vi "Test Find Tests From lvlib.vi"(8 "error in (no error)":errorcluster, 11 "Test Case In":refnum<class "Test FInder Test.lvclass">) -> (0 "error out":errorcluster, 3 "Test Case Out":refnum<class "Test FInder Test.lvclass">)   [LabVIEW 2020, in "Test FInder Test.lvclass"]
uses:
  Test FInder Test.lvclass
  <vilib>/Astemes/LUnit/Test Case.lvclass/Test Case.ctl
  <vilib>/Astemes/LUnit/Core/LUnit Test Case/Private/Append Fail Result.vi
  <vilib>/Astemes/LUnit/Core/LUnit Test Case/Private/Append Pass Result.vi
  <vilib>/Astemes/LUnit/Core/LUnit Test Case/Private/Run In UI.vi
  <vilib>/Utility/error.llb/Clear Errors.vi
  Test FInder Test.lvclass/Test FInder Test.ctl
  source/Framework/Test Finder/Test Finder.lvclass
  source/LUnit Test Suite.lvclass
  80f47747-7e17-4ea4-8ca2-817b5c50055d.vi
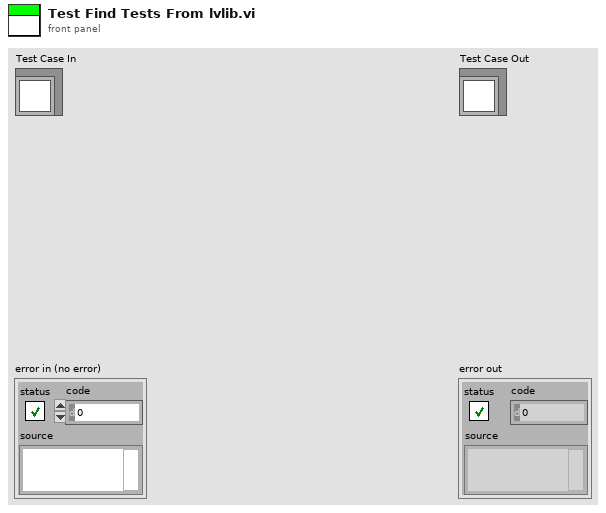
[diagram p1: front panel]
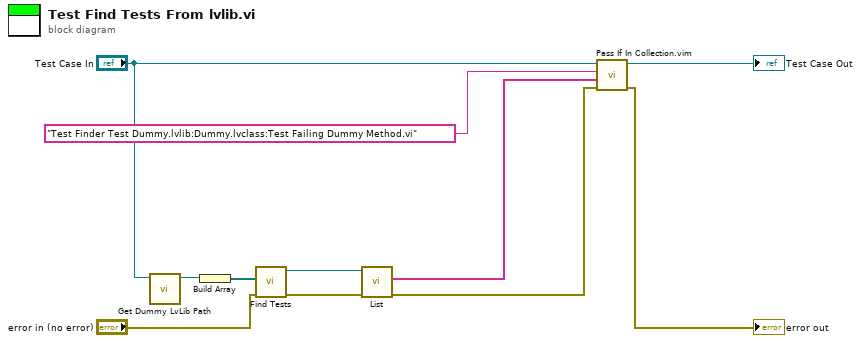
[diagram p0: block diagram]
diagram:
  n1 = call "Get Dummy LvLib Path.vi"("LUnit Test Suite Tests in"="Test Case In") -> ("appended path"=w9:path)  [unwired: 10 in]
  n2 = Build Array(w9) -> (w8:path[])
  n3 = call "Find Tests.vi"("error in (no error)"="error in (no error)", "File Paths"=w8) -> ("error out"=w3:errorcluster, "LUnit Test Suite"=w7:refnum<class "LUnit Test Suite.lvclass">)  [unwired: 8 in]
  n4 = call "List.vi"("error in (no error)"=w3, "LUnit Test Suite In"=w7) -> ("error out"=w2:errorcluster, "List of Runnables"=w4:string[])  [unwired: 8 in]
  n5 = call "Pass If In Collection.vim"("error in (no error)"=w2, "Collection"=w4, "Expected Element"="Test Finder Test Dummy.lvlib:Dummy.lvclass:Test Failing Dummy Method.vi" ("format string"), "LUnit Test Case In"="Test Case In") -> ("error out"=→"error out":errorcluster, "LUnit Test Case Out"=→"Test Case Out":refnum<class "Test FInder Test.lvclass">)  [unwired: 6 in]
